vi "Hex string to AscII string.vi"(4 "hex String":string) -> (1 "ASCII string":string)   [LabVIEW 2013]
doc: "Convert a byte string array (each byte can have any value from 0 to 255) to an ASCII string (twice the length) where each byte is converted into it's corresponding to ASCII characters that represent that number and can be displayed in a string indicator in normal display mode."
panel:
  # "hex display"
  # "normal display"
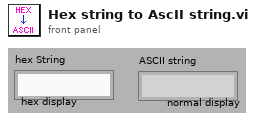
[diagram p1: front panel]
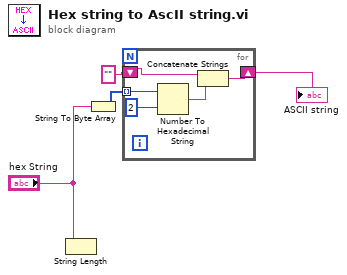
[diagram p0: block diagram]
diagram:
  n1 = String Length(string="hex String") -> ()  [unwired: 1 out]
  n2 = String To Byte Array(string="hex String") -> (unsigned byte array=w3:u8[])
  n3 = for {
    tunnel: w3 -> [w9] mode=indexing
    shift-right: [w6] -> w1
    shift-left: "" -> [w7]
    n4 = Number To Hexadecimal String(1:i16 2 ("width (-)"), 2:w9) -> (0:w8:string)
    n5 = Concatenate Strings(w7, w8) -> (w6:string)
  }
  "ASCII string" <- w1
